vi "Issue Trigger.vi"(8 "error in (no error)":errorcluster, 10 "Channel (1: 1)":i32(ring)=1 items=["1"=1, "2"=2], 11 "VISA resource name":refnum<visa-resource-name>) -> (0 "error out":errorcluster, 3 "VISA resource name out":refnum<visa-resource-name>)   [LabVIEW 2016, in "Agilent 3352X Series.lvlib"]
doc: "Forces an immediate trigger to initiate an arbitrary sequence, sweep, list, or burst for the specified channel. You must first set Trigger Source in the Configure Trigger VI to Software. \nThis VI is intended to be used as an override. For general, software controlled triggering, you should use the Send software Trigger VI.\n\n<b>Note</b>:\n(1) This VI does not check the instrument status. \n(2) If you want to check the instrument status, call the Error Query VI at the conclusion of your sweep operation."
uses:
  Agilent 3352X Series.lvlib
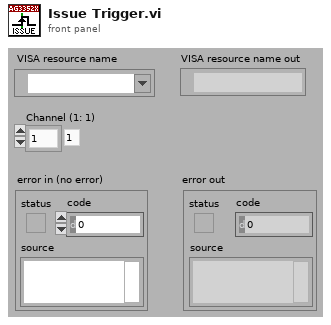
[diagram p1: front panel]
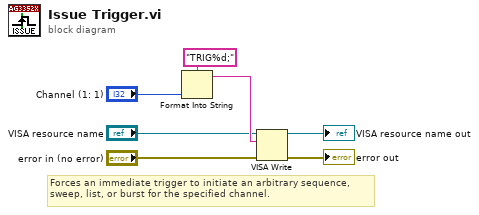
[diagram p0: block diagram]
diagram:
  # "Forces an immediate trigger to initiate an arbitrary sequence, \nsweep, list, or burst for the specified channel."
  n1 = Format Into String(format string="TRIG%d;", "Channel (1: 1)") -> (resulting string=w5:string)  [unwired: 2 in, 1 out]
  n2 = VISA Write(VISA resource name="VISA resource name", write buffer=w5, error in (no error)="error in (no error)") -> (VISA resource name out=→"VISA resource name out":refnum<visa-resource-name>, error out=→"error out":errorcluster)  [unwired: 1 out]
